vi "Write Queue Properties.vi"(8 "error in (no error)":errorcluster, 10 "Queue Properties":T1={"Number of Queues (3)"=3, "Create Queue References? (F)"=FALSE, "Max Queue Sizes (-1, unlimited)"=[-1, 1, 1]}, 11 "ModuleAdmin in":refnum<class "ModuleAdmin.lvclass">) -> (0 "error out":errorcluster, 3 "ModuleAdmin out":refnum<class "ModuleAdmin.lvclass">)   [LabVIEW 2018, in "ModuleAdmin.lvlib" / "ModuleAdmin.lvclass"]
uses:
  ModuleAdmin.lvclass
  TypeDefinitions/QueueProperties.ctl
  ModuleAdmin.lvclass/ModuleAdmin.ctl
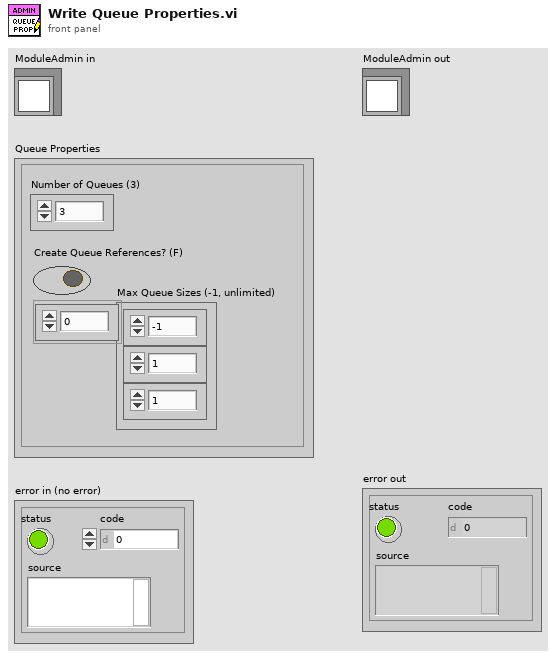
[diagram p1: front panel]
types:
  T1 = typedef "ModuleAdmin.lvlib/ModuleAdmin.lvclass/QueueProperties.ctl" = cluster{"Number of Queues (3)":i32, "Create Queue References? (F)":bool, "Max Queue Sizes (-1, unlimited)":i32[]}
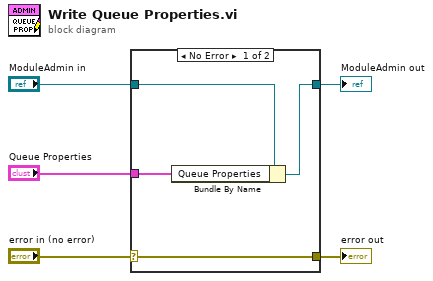
[diagram p0: block diagram]
diagram:
  n1 = case shown="No Error" "error in (no error)" {
    selector: "error in (no error)" -> [w9 w10]
    tunnel: [w9 w10] -> w4
    tunnel: [w7 w11] -> w2
    tunnel: "ModuleAdmin in" -> [w8 w11]
    tunnel: "Queue Properties" -> [w6 _]
    frame No Error {
      n2 = Bundle By Name(cluster=w8, "Queue Properties"=w6) -> (w7:refnum<class "ModuleAdmin.lvclass">)
    }
    frame Error {
    }
  }
  "error out" <- w4
  "ModuleAdmin out" <- w2
